vi "Lab_Temp_PID.vi"(1 "Valve Pos":dbl format="%.2f", 2 "Previous Control Sum":dbl format="%.2f", 3 "Present Value":dbl=15.0 format="%.2f", 4 "Setpoint":dbl=15.0 format="%.2f") -> (0 "Dem Output":dbl format="%.2f")   [LabVIEW 2015]
uses:
  <vilib>/Analysis/NI_AALPro.lvlib
panel:
  in  "O/P deadband":dbl format="%.2f"
  in  "Kp Deadband":dbl format="%.2f"
  in  "Derivative History":i32=20
  out "deadbanded error":dbl format="%.2f"
  in  "P":bool=TRUE
  in  "D":bool=TRUE
  in  "I":bool=TRUE
  out "Waveform Chart":T1(graph)
  in  "Manual Demand":dbl min=-100.0 max=100.0 format="%.2f"
  in  "Manual Override":bool
  out "Control Sum":dbl format="%.2f"
  out "Derivative Term":dbl format="%.2f"
  out "Integral Term":dbl format="%.2f"
  out "error differential":dbl format="%.5f"
  out "Proportional Term":dbl format="%.2f"
  in  "Kd":dbl=50.0 format="%.2f"
  in  "Ki":dbl=0.025 format="%.3f"
  in  "Kp":dbl=30.0 format="%.2f"
  out "error":dbl format="%.2f"
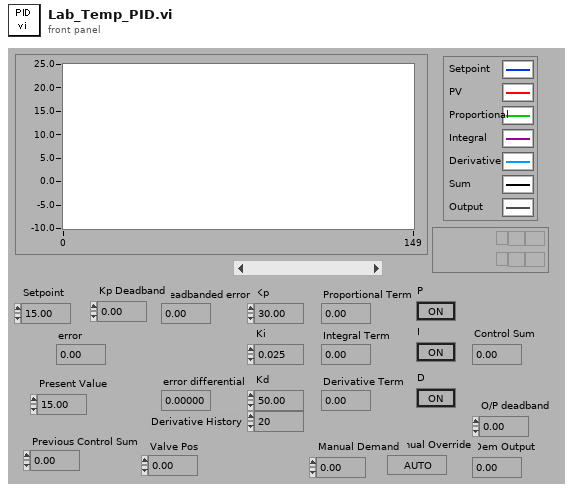
[diagram p1: front panel]
types:
  T1 = cluster{"Setpoint":dbl, "Present Value":dbl, "Proportional Term":dbl, "Integral Term":dbl, "Derivative Term":dbl, "Control Sum":dbl, "Dem Output":dbl}
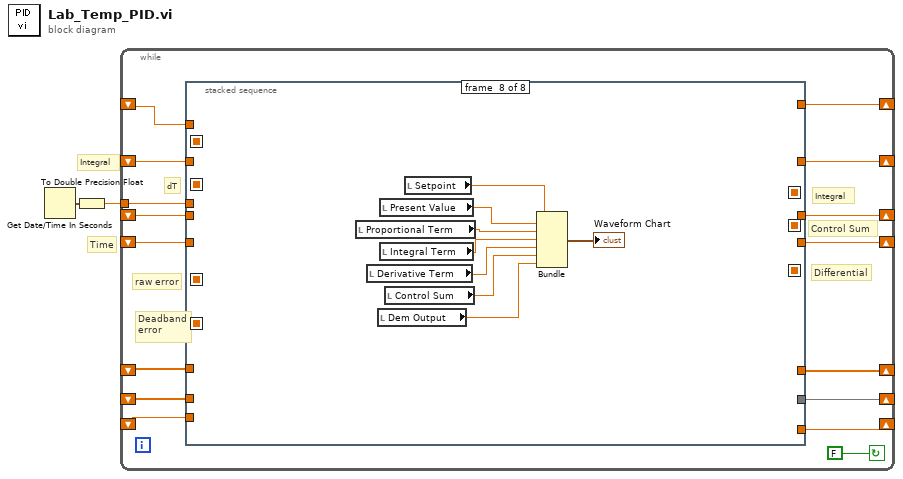
[diagram p0: block diagram]
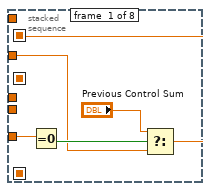
[diagram p2: hidden frame]
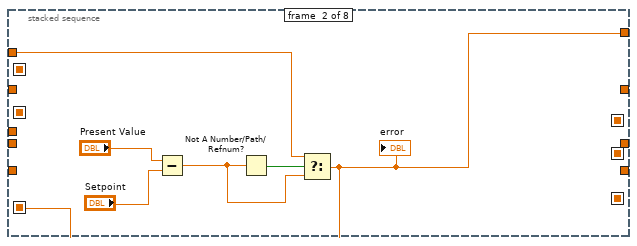
[diagram p3: hidden frame]
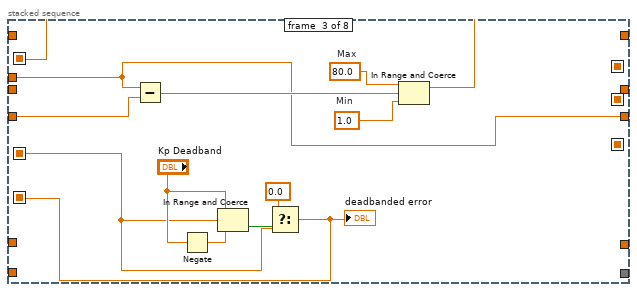
[diagram p4: hidden frame]
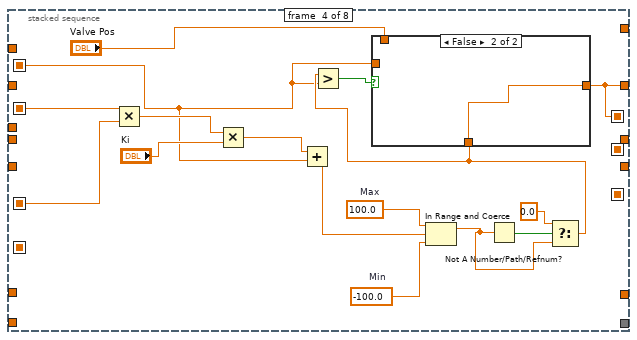
[diagram p5: hidden frame]
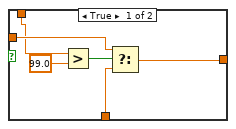
[diagram p6: hidden frame]
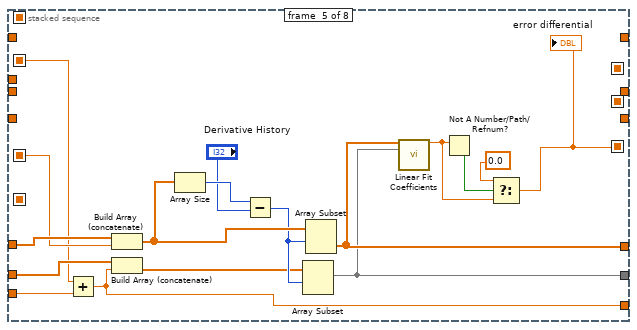
[diagram p7: hidden frame]
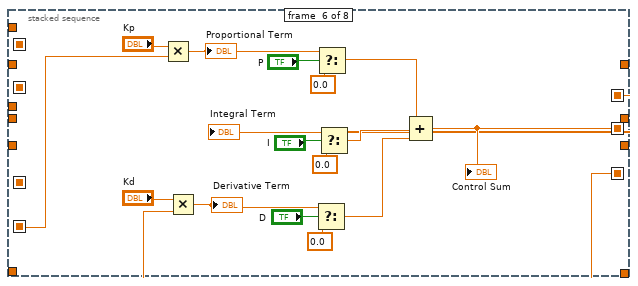
[diagram p8: hidden frame]
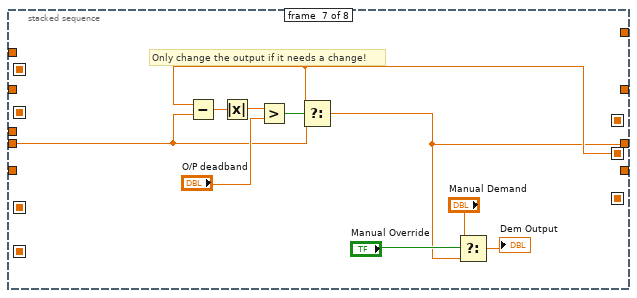
[diagram p9: hidden frame]
diagram:
  # "Integral"
  # "Time"
  n1 = Get Date/Time In Seconds() -> (seconds since 1Jan1904=w1:timestamp)
  n2 = To Double Precision Float(number=w1) -> (double precision float=w2:dbl)
  n3 = while {
    shift-left: _ -> [w5]
    shift-right: [w4] -> _
    shift-left: _ -> [w7]
    shift-right: [w6] -> _
    shift-left: _ -> [w9]
    shift-right: [w8] -> _
    tunnel: w2 -> [w14]
    shift-left: _ -> [w11]
    shift-right: [w10] -> _
    shift-left: _ -> [w13]
    shift-right: [w12] -> _
    shift-left: _ -> [w15]
    shift-right: [w16] -> _
    shift-left: _ -> [w18]
    shift-right: [w17] -> _
    stop <- FALSE continue-if-true
    # "Control Sum"
    # "raw error"
    # "Differential"
    # "Integral"
    # "Deadband\nerror"
    # "dT"
    n4 = stacked-sequence {
      seq-local: [_ _ w30 _ _ _ _ _] -> [_ _ _ w57 w67 _ _ _]
      seq-local: [_ _ w39 _ _ _ _ _] -> [_ _ _ _ _ w84 _ _]
      seq-local: [_ _ _ _ w72 _ _ _] -> [_ _ _ _ _ w83 _ _]
      seq-local: [_ _ _ w43 _ _ _ _] -> [_ _ _ _ _ w82 _ _]
      seq-local: [_ w25 _ _ _ _ _ _] -> [_ _ w31 w55 w73 _ _ _]
      seq-local: [_ _ _ _ _ w87 _ _] -> [_ _ _ _ _ _ w102 _]
      seq-local: [w19 _ _ _ _ _ _ _] -> [_ _ _ w42 _ _ _ _]
      tunnel: w18 -> [w23 _ w36 _ _ _ _ _]
      tunnel: [_ _ w34 _ _ _ _ _] -> w17
      tunnel: [_ _ _ w43 _ _ _ _] -> w16
      tunnel: w15 -> [w20 _ _ _ _ _ _ _]
      tunnel: w14 -> [_ _ w34 _ _ _ _ _]
      tunnel: w13 -> [_ _ _ _ w81 _ _ _]
      tunnel: [_ _ _ _ w74 _ _ _] -> w12
      tunnel: w11 -> [_ _ _ _ w80 _ _ _]
      tunnel: [_ _ _ _ w71 _ _ _] -> w10
      tunnel: w9 -> [_ _ _ _ _ _ w100 _]
      tunnel: [_ _ _ _ _ _ w99 _] -> w8
      tunnel: w7 -> [_ _ _ _ w66 _ _ _]
      tunnel: [_ _ _ _ w65 _ _ _] -> w6
      tunnel: w5 -> [_ w26 _ _ _ _ _ _]
      tunnel: [_ w25 _ _ _ _ _ _] -> w4
      frame #0 {
        n5 = Equal To 0?(x=w23) -> (x = 0?=w22:bool)
        n6 = Select(t="Previous Control Sum", s=w22, f=w20) -> (s? t:f=w19:dbl)
      }
      frame #1 {
        n7 = Subtract(x="Present Value", y="Setpoint") -> (x-y=w24:dbl)
        n8 = Not A Number/Path/Refnum?(number/path/refnum=w24) -> (NaN/Path/Refnum?=w27:bool)
        n9 = Select(t=w26, s=w27, f=w24) -> (s? t:f=w25:dbl)
        "error" <- w25
      }
      frame #2 {
        w37 = 1.0  # Min
        w38 = 80.0  # Max
        n10 = Subtract(x=w34, y=w36) -> (x-y=w35:dbl)
        n11 = Negate(x="Kp Deadband") -> (-x=w33:dbl)
        n12 = In Range and Coerce(upper limit="Kp Deadband", x=w31, lower limit=w33) -> (In Range?=w40:bool)  [unwired: 1 out]
        n13 = Select(t=0.0, s=w40, f=w31) -> (s? t:f=w39:dbl)
        "deadbanded error" <- w39
        n14 = In Range and Coerce(upper limit=w38, x=w35, lower limit=w37) -> (coerced(x)=w30:dbl)  [unwired: 1 out]
      }
      frame #3 {
        w47 = -100.0  # Min
        w48 = 100.0  # Max
        n15 = Multiply(x=w57, y=w55) -> (x*y=w51:dbl)
        n16 = Multiply(x=w51, y="Ki") -> (x*y=w49:dbl)
        n17 = Add(x=w49, y=w42) -> (x+y=w56:dbl)
        n18 = In Range and Coerce(upper limit=w48, x=w56, lower limit=w47) -> (coerced(x)=w53:dbl)  [unwired: 1 out]
        n19 = Not A Number/Path/Refnum?(number/path/refnum=w53) -> (NaN/Path/Refnum?=w54:bool)
        n20 = Select(t=0.0, s=w54, f=w53) -> (s? t:f=w45:dbl)
        n21 = Greater?(x=w45, y=w42) -> (0:w46:bool)
        n22 = case shown="False" w46 {
          tunnel: w45 -> [w63 w64]
          tunnel: w42 -> [w62 _]
          tunnel: [w61 w64] -> w43
          tunnel: "Valve Pos" -> [w59 _]
          frame True {
            n23 = Greater?(x=w59, y=99.0) -> (0:w58:bool)
            n24 = Select(t=w62, s=w58, f=w63) -> (s? t:f=w61:dbl)
          }
          frame False {
          }
        }
      }
      frame #4 {
        n25 = Add(x=w67, y=w66) -> (x+y=w65:dbl)
        n26 = Build Array (concatenate)(w81, w73) -> (w77:dbl[])
        n27 = Build Array (concatenate)(w80, w65) -> (w75:dbl[])
        n28 = Array Size(array=w77) -> (size(s)=w79:i32)
        n29 = Subtract(x=w79, y="Derivative History") -> (x-y=w76:i32)
        n30 = Array Subset(array=w75, index=w76) -> (w71:dbl[])  [unwired: 1 in]
        n31 = Array Subset(array=w77, index=w76) -> (w74:dbl[])  [unwired: 1 in]
        n32 = call <vilib>:"Linear Fit Coefficients.vi"("Y"=w74, "X"=w71) -> ("slope"=w68:dbl)  [unwired: 3 in, 10 out]
        n33 = Not A Number/Path/Refnum?(number/path/refnum=w68) -> (NaN/Path/Refnum?=w70:bool)
        n34 = Select(t=0.0 ("f"), s=w70, f=w68) -> (s? t:f=w72:dbl)
        "error differential" <- w72
      }
      frame #5 {
        n35 = Multiply(x="Kp", y=w84) -> (x*y=w96:dbl)
        "Proportional Term" <- w96
        n36 = Multiply(x="Kd", y=w83) -> (x*y=w88:dbl)
        "Derivative Term" <- w88
        n37 = Select(t=w88, s="D", f=0.0) -> (s? t:f=w90:dbl)
        n38 = Select(t=w96, s="P", f=0.0) -> (s? t:f=w97:dbl)
        n39 = Select(t=w82, s="I", f=0.0) -> (s? t:f=w89:dbl)
        n40 = Compound Arithmetic op=ADD(w97, w89, w90) -> (w87:dbl)
        "Control Sum" <- w87
        "Integral Term" <- w82
      }
      frame #6 {
        # "Only change the output if it needs a change!"
        n41 = Subtract(x=w102, y=w100) -> (x-y=w105:dbl)
        n42 = Absolute Value(x=w105) -> (abs(x)=w104:dbl)
        n43 = Greater?(x=w104, y="O/P deadband") -> (0:w103:bool)
        n44 = Select(t=w102, s=w103, f=w100) -> (s? t:f=w99:dbl)
        n45 = Select(t="Manual Demand", s="Manual Override", f=w99) -> (s? t:f=→"Dem Output":dbl)
      }
      frame #7 {
        n46 = local read "Proportional Term"() -> (w112:dbl)
        n47 = local read "Derivative Term"() -> (w114:dbl)
        n48 = local read "Dem Output"() -> (w116:dbl)
        n49 = local read "Present Value"() -> (w111:dbl)
        n50 = local read "Integral Term"() -> (w113:dbl)
        n51 = local read "Control Sum"() -> (w115:dbl)
        n52 = local read "Setpoint"() -> (w110:dbl)
        n53 = Bundle("Setpoint"=w110, "Present Value"=w111, "Proportional Term"=w112, "Integral Term"=w113, "Derivative Term"=w114, "Control Sum"=w115, "Dem Output"=w116) -> (→"Waveform Chart":T1)  [unwired: 1 out]
      }
    }
  }
